vi "SeedFeeder.vi"() -> ()   [LabVIEW 2018]
uses:
  <resource>/objmgr/daqmx.rc
  <vilib>/Analysis/NI_AALPro.lvlib
panel:
  out "Arithmetic Mean":dbl(slide) scale=0.0..2000.0
  in  "milliseconds to wait":u32=250
  out "M (seed)":cluster{"X":dbl[], "Y":dbl[]}[](graph)
  out "dM/dt (seed)":cluster{"X":dbl[], "Y":dbl[]}(graph)
  in  "stop":bool
  in  "Currents Task Name":refnum<k21>="TestCurrents"
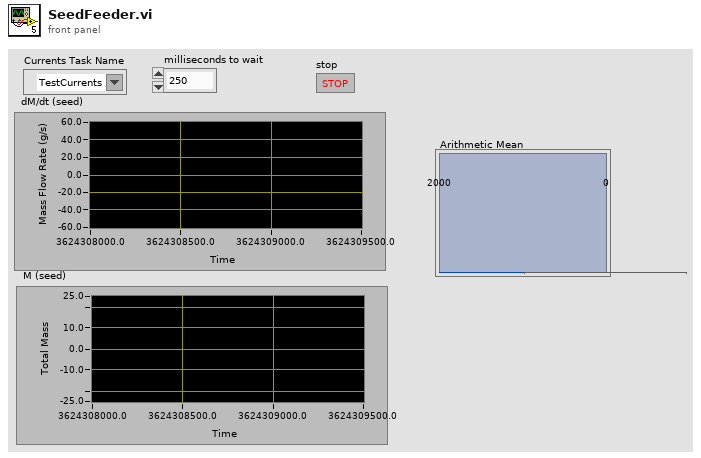
[diagram p1: front panel]
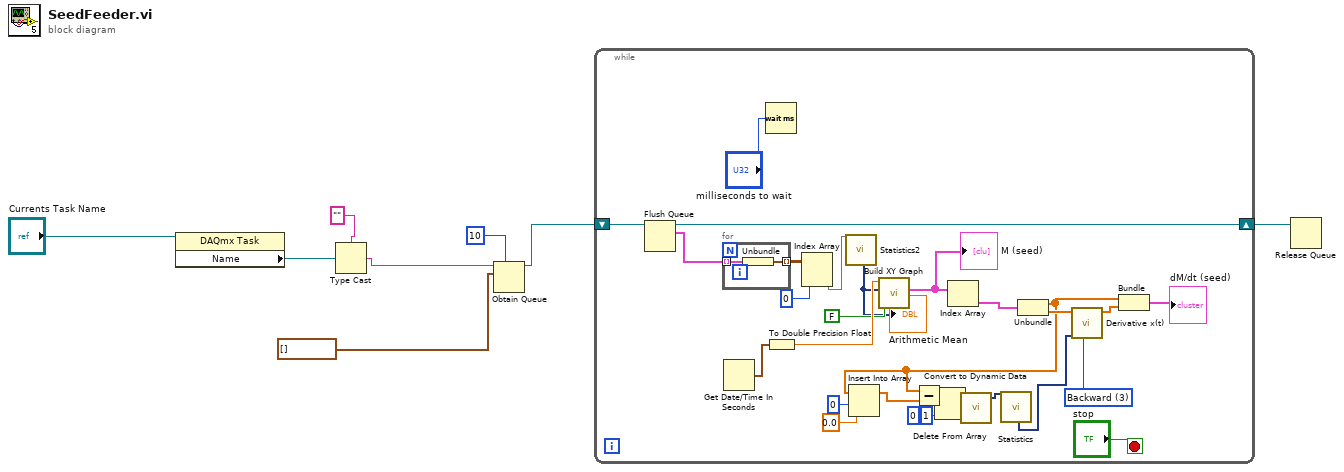
[diagram p0: block diagram]
diagram:
  n1 = property class="DAQmx Task"(reference="Currents Task Name") -> ("Name"=w8:refnum<k21>)  [unwired: 1 in, 2 out]
  n2 = Type Cast(type="", x=w8) -> (*(type *) &x=w7:string)
  n3 = Obtain Queue(max queue size (-1, unlimited)=10, name (unnamed)=w7, element data type=waveform(dbl)[] [] ("data")) -> (queue out=w2:refnum<queue>)  [unwired: 2 in, 2 out]
  n4 = while {
    shift-right: [w34] -> w1
    shift-left: w2 -> [w36]
    stop <- "stop" stop-if-true
    w26 = u16 3 items=["2nd Order Central", "4th Order Central", "Forward", "Backward"] ("method")
    n5 = Flush Queue(queue=w36) -> (queue out=w34:refnum<queue>, remaining elements=w35:cluster{"data":waveform(dbl)[]}[])  [unwired: 1 in, 1 out]
    n6 = for {
      tunnel: w35 -> [w38] mode=indexing
      tunnel: [w37] -> w33 mode=indexing
      n7 = Unbundle(w38) -> ("data"=w37:waveform(dbl)[])
    }
    n8 = Get Date/Time In Seconds() -> (seconds since 1Jan1904=w32:timestamp)
    n9 = Wait (ms)(milliseconds to wait="milliseconds to wait") -> ()  [unwired: 1 out]
    n10 = To Double Precision Float(number=w32) -> (double precision float=w31:dbl)
    n11 = Index Array(array=w33, index (col)=0 ("index (row)")) -> (element=w16:waveform(dbl)[])  [unwired: 1 in]
    n12 = call "Statistics2"("Signals"=w16) -> ("Arithmetic Mean"=w15:dynamicdata)  [unwired: 25 in, 1 out]
    "Arithmetic Mean" <- w15
    n13 = call "Build XY Graph"("Reset"=FALSE, "Y Input"=w15, "X Input"=w31) -> ("XY Graph"=w14:cluster{"X":dbl[], "Y":dbl[]}[])  [unwired: 7 in, 1 out]
    "M (seed)" <- w14
    n14 = Index Array(array=w14) -> (element=w28:cluster{"X":dbl[], "Y":dbl[]})  [unwired: 1 in]
    n15 = Unbundle(w28) -> ("X"=w10:dbl[], "Y"=w27:dbl[])
    n16 = Insert Into Array(array=w10, index=0, new element=0.0 ("new element/subarray")) -> (w9:dbl[])
    n17 = Subtract(x=w10, y=w9) -> (x-y=w23:dbl[])
    n18 = Delete From Array(array=w23, length=1, index=0) -> (array with subset deleted=w13:dbl[])  [unwired: 1 out]
    n19 = call "Convert to Dynamic Data"("Array"=w13) -> ("Dynamic Data Type"=w22:dynamicdata)  [unwired: 3 in]
    n20 = call "Statistics"("Signals"=w22) -> ("Arithmetic Mean"=w21:dynamicdata)  [unwired: 25 in, 1 out]
    n21 = call <vilib>:"Derivative x(t).vi"("method"=w26, "dt"=w21, "X"=w27) -> ("dX/dt"=w25:dbl[])  [unwired: 7 in, 1 out]
    n22 = Bundle("X"=w10, "dX/dt"=w25) -> (→"dM/dt (seed)":cluster{"X":dbl[], "dX/dt":dbl[]})  [unwired: 1 in]
  }
  n23 = Release Queue(queue=w1) -> ()  [unwired: 2 in, 3 out]
